vi "raise stop recieve.vi"(8 "error in (no error)":errorcluster, 11 "y":bool) -> (0 "error out":errorcluster, 2 "Stop_state":bool)   [LabVIEW 2019]
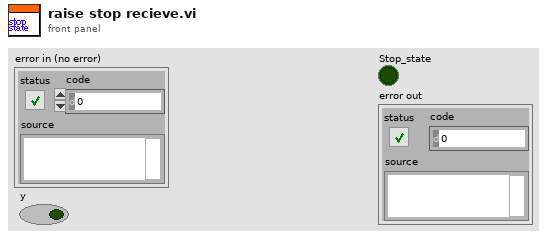
[diagram p1: front panel]
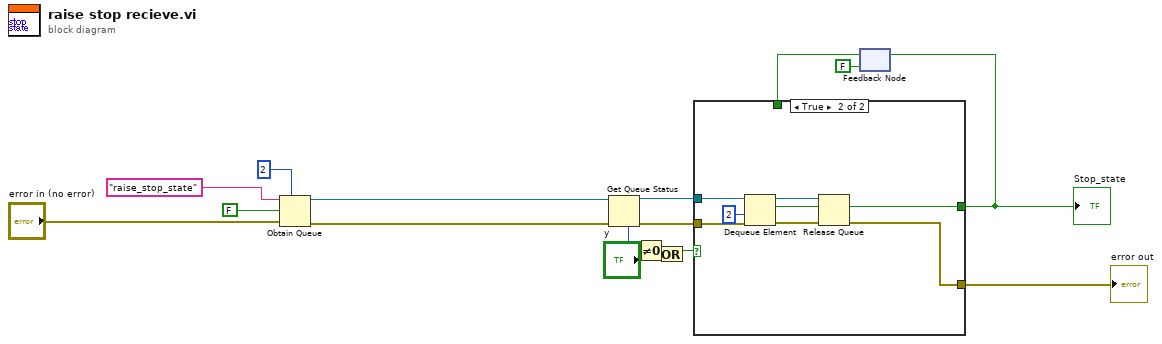
[diagram p0: block diagram]
diagram:
  n1 = Obtain Queue(max queue size (-1, unlimited)=2, name (unnamed)="raise_stop_state", element data type=FALSE, error in (no error)="error in (no error)") -> (queue out=w11:refnum<queue>, error out=w12:errorcluster)  [unwired: 1 in, 1 out]
  n2 = Get Queue Status(queue=w11, error in (no error)=w12) -> (queue out=w8:refnum<queue>, error out=w7:errorcluster, # elements in queue=w10:i32)  [unwired: 1 in, 5 out]
  n3 = Not Equal To 0?(x=w10) -> (x != 0?=w9:bool)
  n4 = Or(x=w9, y="y") -> (x .or. y?=w2:bool)
  n5 = feedback #1(FALSE) -> (w5:bool)
  n6 = case shown="True" w2 {
    tunnel: w8 -> [_ w25]
    tunnel: w7 -> [w17 w24]
    tunnel: [w18 w23] -> w6
    tunnel: w5 -> [w18 _]
    tunnel: [w17 w21] -> w4
    frame False {
    }
    frame True {
      n7 = Dequeue Element(queue=w25, timeout in ms (-1)=2, error in (no error)=w24) -> (queue out=w20:refnum<queue>, element=w23:bool, error out=w22:errorcluster)  [unwired: 1 out]
      n8 = Release Queue(queue=w20, error in (no error)=w22) -> (error out=w21:errorcluster)  [unwired: 1 in, 2 out]
    }
  }
  "Stop_state" <- w6
  "error out" <- w4
  n9 = feedback-in #1(w6) -> ()
